vi "Update_UI.vi"(8 "error in (no error)":errorcluster, 10 "srcsettings":T1, 11 "IB_Settings_Item_Destination in":refnum<class "IB_Settings_Item_Destination.lvclass">) -> (0 "error out":errorcluster, 2 "validate permisions?":bool, 3 "IB_Settings_Item_Destination out":refnum<class "IB_Settings_Item_Destination.lvclass">)   [LabVIEW 2020, in "IB_Settings_Item_Destination.lvclass"]
uses:
  <vilib>/AppBuilder/IB_Classes/Settings_Item_Destination/IB_Settings_Item_Destination.lvclass
  <vilib>/AppBuilder/IB_Classes/Settings_Item_Destination/IB_Settings_Item_Destination.lvclass/IB_Settings_Item_Destination.ctl
  <vilib>/AppBuilder/IB_Classes/Settings_Item/IB_Settings_Item.lvclass
  e:/builds/penguin/labview/branches/2020/dev/dist/vi.lib/AppBuilder/IB_Classes/Settings_Item/IB_Settings_Item.lvclass
  e:/builds/penguin/labview/branches/2020/dev/dist/vi.lib/AppBuilder/IB_Classes/Settings_Item_Destination/IB_Settings_Item_Destination.lvclass
  <resource>/Framework/Providers/Builds/Installer/CDK_sTypeDef_FILEATTRIBUTES.ctl
  <resource>/Framework/Providers/Builds/Installer/Pages/controls/IB_UI_Page_SrcSettings_References.ctl
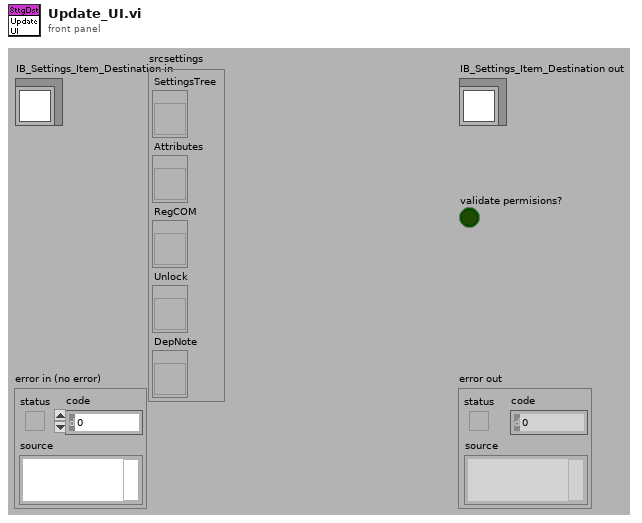
[diagram p1: front panel]
types:
  T1 = typedef "IB_UI_Page_SrcSettings_References.ctl" = cluster{"SettingsTree":refnum<vi>, "Attributes":refnum<vi>, "RegCOM":refnum<vi>, "Unlock":refnum<vi>, "DepNote":refnum<vi>}
  T2 = typedef "IB_Settings_Item.ctl" = cluster{"address":string[], "Attributes":i16, "RegCOM":bool, "unlock":bool}
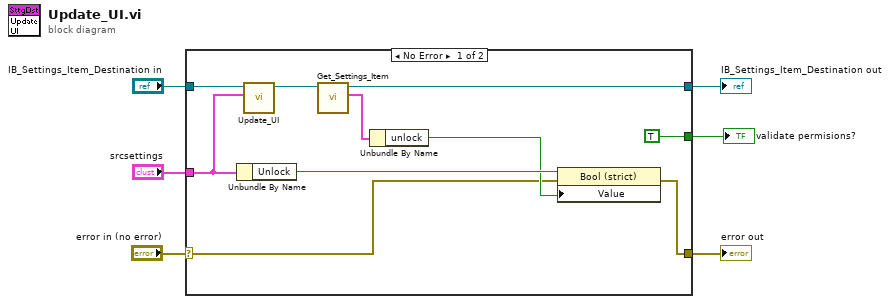
[diagram p0: block diagram]
diagram:
  n1 = case shown="No Error" "error in (no error)" {
    selector: "error in (no error)" -> [w9 w18]
    tunnel: [w8 w18] -> w5
    tunnel: "srcsettings" -> [w14 _]
    tunnel: "IB_Settings_Item_Destination in" -> [w13 w17]
    tunnel: [w16 w17] -> w2
    tunnel: [TRUE _] -> w1
    frame No Error {
      n2 = Unbundle By Name(w14) -> ("Unlock"=w15:refnum<vi>)
      n3 = call-parent "Update_UI.vi"("srcsettings"=w14, "IB_Settings_Item in"=w13) -> ("IB_Settings_Item out"=w12:refnum<class "IB_Settings_Item_Destination.lvclass">)  [unwired: 7 in, 2 out]
      n4 = call <vilib>:"Get_Settings_Item.vi"("IB_Settings_Item in"=w12) -> ("data"=w11:T2, "IB_Settings_Item out"=w16:refnum<class "IB_Settings_Item_Destination.lvclass">)  [unwired: 8 in, 1 out]
      n5 = Unbundle By Name(w11) -> ("unlock"=w10:bool)
      n6 = property class="Bool (strict)"(reference=w15, error in=w9, "Value"=w10) -> (error out=w8:errorcluster)  [unwired: 1 out]
    }
    frame Error {
    }
  }
  "error out" <- w5
  "IB_Settings_Item_Destination out" <- w2
  "validate permisions?" <- w1
